vi "DriveAndLiftAndIntake.vi"(6 "Intake Time":dbl, 7 "First Iteration":bool, 8 "Intake Select":dbl, 9 "Level":dbl, 10 "Distance":dbl, 11 "Speed":dbl) -> (0 "Done?":bool, 2 "Joy Y":dbl, 3 "Joy X":dbl)   [LabVIEW 2014]
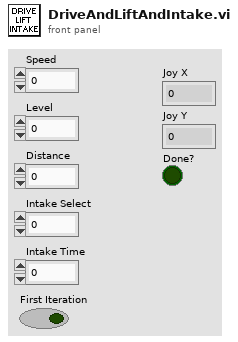
[diagram p1: front panel]
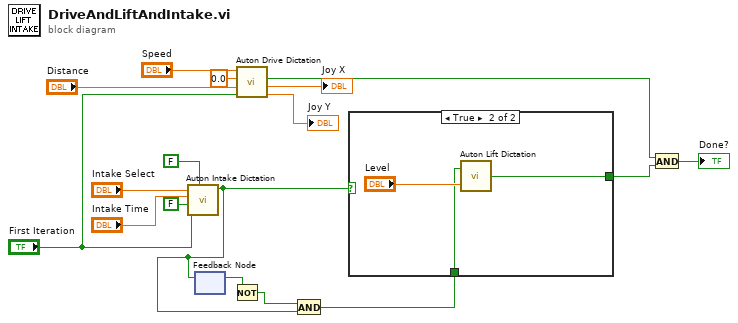
[diagram p0: block diagram]
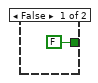
[diagram p2: hidden frame]
diagram:
  n1 = call "Auton Intake Dictation.vi"("Roller Arms In"=FALSE, "First Iteration"="First Iteration", "Roller Arms Same"=FALSE, "Time"="Intake Time", "Intake Select"="Intake Select") -> ("Time has Elapsed"=w11:bool)  [unwired: 6 in]
  n2 = feedback #1() -> (w13:bool)  [unwired: 1 in]
  n3 = feedback-in #1(w11) -> ()
  n4 = Not(x=w13) -> (.not. x?=w12:bool)
  n5 = call "Auton Drive Dictation.vi"("Reset Encoders"="First Iteration", "Distance (inches)"="Distance", "Direction (0-359)"=0.0, "Speed (-1 to 1)"="Speed") -> ("Joy Y"=→"Joy Y":dbl, "Joy X"=→"Joy X":dbl, "Distance Reached?"=w8:bool)  [unwired: 5 in]
  n6 = And(x=w12, y=w11) -> (x .and. y?=w10:bool)
  n7 = case shown="True" w11 {
    tunnel: w10 -> [_ w20]
    tunnel: [FALSE ("Lift Sequence Done") w19] -> w9
    frame False {
    }
    frame True {
      n8 = call "Auton Lift Dictation.vi"("Level"="Level", "First Iteration"=w20) -> ("Lift Sequence Done"=w19:bool)
    }
  }
  n9 = And(x=w8, y=w9) -> (x .and. y?=→"Done?":bool)
